vi "HandleAlarms.vi"(0 "reference in":refnum<class "AI.lvclass">, 11 "error in (no error)":errorcluster) -> (4 "reference out":refnum<class "AI.lvclass">, 15 "error out":errorcluster)   [LabVIEW 2019, in "AI.lvclass"]
uses:
  AI.lvclass
  AI.lvclass/AI.ctl
  AnalogComparator_class/AnalogComparator.lvclass/AnalogComparator.ctl
  AnalogComparator_class/SendToDb.vi
  AnalogComparator_class/AnalogComparator.lvclass
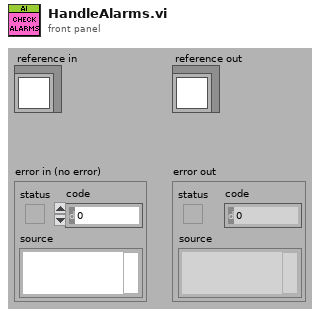
[diagram p1: front panel]
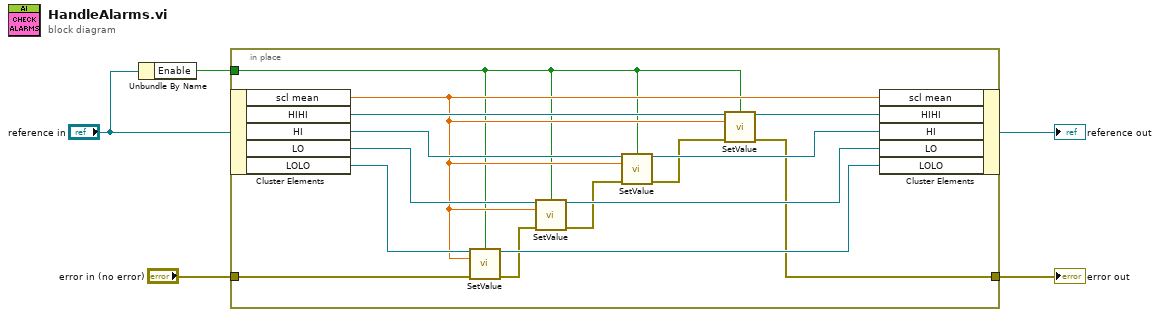
[diagram p0: block diagram]
diagram:
  n1 = Unbundle By Name("reference in") -> ("Enable"=w1:bool)
  n2 = in-place {
    in-place-border: [w8] -> w4
    in-place-border: "error in (no error)" -> [w7]
    in-place-border: w1 -> [w6]
    n3 = in-place-cluster #1("reference in") -> ("scl mean"=w12:dbl, "HIHI"=w20:refnum<class "AnalogComparator.lvclass">, "HI"=w18:refnum<class "AnalogComparator.lvclass">, "LO"=w16:refnum<class "AnalogComparator.lvclass">, "LOLO"=w14:refnum<class "AnalogComparator.lvclass">)
    n4 = call "SetValue.vi"("class data in"=w14, "Enable"=w6, "Value"=w12, "error in (no error)"=w7) -> ("class data out"=w13:refnum<class "AnalogComparator.lvclass">, "error out"=w11:errorcluster)  [unwired: 10 in]
    n5 = call "SetValue.vi"("class data in"=w16, "Enable"=w6, "Value"=w12, "error in (no error)"=w11) -> ("class data out"=w15:refnum<class "AnalogComparator.lvclass">, "error out"=w10:errorcluster)  [unwired: 10 in]
    n6 = call "SetValue.vi"("class data in"=w18, "Enable"=w6, "Value"=w12, "error in (no error)"=w10) -> ("class data out"=w17:refnum<class "AnalogComparator.lvclass">, "error out"=w9:errorcluster)  [unwired: 10 in]
    n7 = call "SetValue.vi"("class data in"=w20, "Enable"=w6, "Value"=w12, "error in (no error)"=w9) -> ("class data out"=w19:refnum<class "AnalogComparator.lvclass">, "error out"=w8:errorcluster)  [unwired: 10 in]
    n8 = in-place-cluster #1("scl mean"=w12, "HIHI"=w19, "HI"=w17, "LO"=w15, "LOLO"=w13) -> (→"reference out":refnum<class "AI.lvclass">)
  }
  "error out" <- w4
